vi "Get Test Index Location.vi"(8 "error in (no error)":errorcluster) -> (0 "error out":errorcluster, 3 "Test Index Location":path)   [LabVIEW 2020, in "Execution API.lvclass"]
uses:
  Execution API.lvclass
  <vilib>/Utility/sysdir.llb/System Directory Type.ctl
  Execution API.lvclass/Execution API.ctl
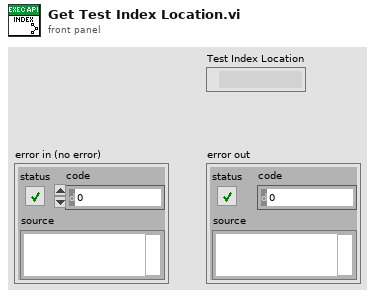
[diagram p1: front panel]
types:
  T1 = typedef "System Directory Type.ctl" = i32
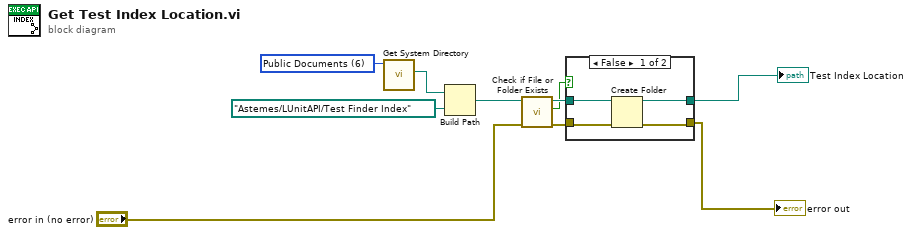
[diagram p0: block diagram]
diagram:
  w5 = T1 6 items=["User Home"=0, "User Desktop"=1, "User Documents"=2, "User Application Data"=3, "User Preferences"=4, "User Temporary"=5, "Public Documents"=6, "Public Application Data"=7, "Public Preferences"=8, "Public Cache"=13, "System Core Libraries"=9, "System Installed Libraries"=10, "Application Files"=11, "Boot Volume Root"=12] ("system directory type")
  n1 = call <vilib>:"Get System Directory.vi"("system directory type"=w5) -> ("system directory"=w7:path)  [unwired: 10 in]
  n2 = Build Path(base path=w7, name or relative path=path "Astemes/LUnitAPI/Test Finder Index") -> (appended path=w4:path)
  n3 = call <vilib>:"Check if File or Folder Exists.vi"("error in (no error)"="error in (no error)", "path"=w4) -> ("error out"=w2:errorcluster, "file or folder exists?"=w1:bool, "dup path"=w3:path)  [unwired: 7 in]
  n4 = case shown="False" w1 {
    tunnel: [w12 w15] -> w8
    tunnel: [w11 w16] -> w10
    tunnel: w3 -> [w14 w16]
    tunnel: w2 -> [w13 w15]
    frame False {
      n5 = Create Folder(path (use dialog)=w14, error in=w13) -> (created path=w11:path, error out=w12:errorcluster)  [unwired: 1 in, 1 out]
    }
    frame True {
    }
  }
  "Test Index Location" <- w10
  "error out" <- w8
